vi "AlignProc.vi"(10 "BCGT":T1={"Brightness"=171.0, "Contrast"=89.0, "Gamma"=2.0, "Threshold_Low"=0.0, "Threshold_High"=144.0} {"Threshold_High" min=0.0 max=255.0 step=1.0 scale=0.0..255.0; "Threshold_Low" min=0 max=255 step=1 scale=0.0..255.0 scale format="%.2f"; "Gamma" min=0.1 max=10 step=0.01 scale=0.1..10.0 scale format="%.1f"; "Contrast" min=1 max=89 step=0.1 scale=0.0..89.0 scale format="%.2f"; "Brightness" min=0 max=255 step=1 scale=0.0..255.0 scale format="%.2f"}, 11 "Img_In":T2(plugin-control)) -> (0 "Distances":sgl[](array[numeric]) format="%.4f", 1 "Number of Particles":i32, 2 "Boolean":bool, 3 "Image Out":T2(plugin-control), 4 "Array":cluster{"Numeric":dbl, "Numeric":dbl}[](array[cluster]))   [LabVIEW 2013]
uses:
  <vilib>/Analysis/baseanly.llb/Mean (DBL).vi
  <vilib>/Analysis/NI_AALBase.lvlib
  <vilib>/vision/NI_Vision_Development_Module.lvlib
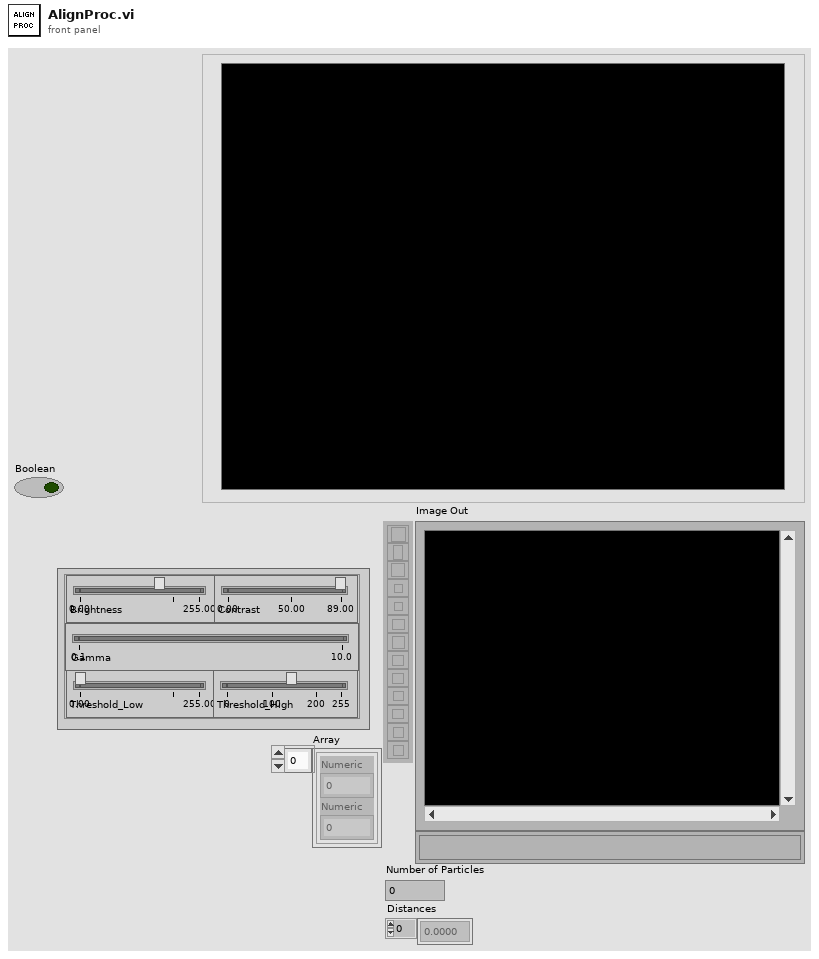
[diagram p1: front panel]
types:
  T1 = cluster{"Brightness":sgl, "Contrast":sgl, "Gamma":sgl, "Threshold_Low":sgl, "Threshold_High":dbl}
  T2 = typedef "IMAQ Image.ctl" = refnum<image>
  T3 = cluster{"Brightness":sgl, "Contrast":sgl, "Gamma":sgl}
  T4 = cluster{"Threshold_Low":sgl, "Threshold_High":dbl}
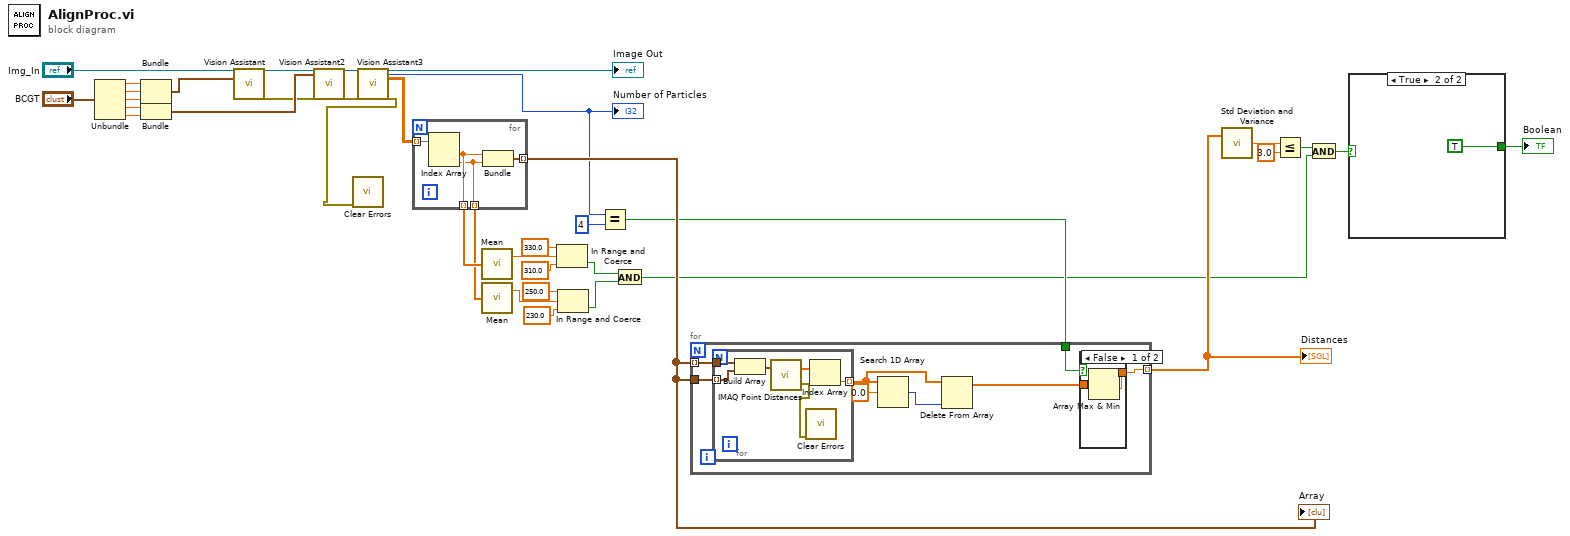
[diagram p0: block diagram]
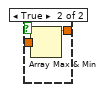
[diagram p2: hidden frame]
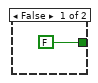
[diagram p3: hidden frame]
diagram:
  n1 = Unbundle("BCGT") -> ("Brightness"=w35:sgl, "Contrast"=w34:sgl, "Gamma"=w33:sgl, "Threshold_Low"=w31:sgl, "Threshold_High"=w30:dbl)
  n2 = Bundle("Brightness"=w35, "Contrast"=w34, "Gamma"=w33) -> (w32:T3)  [unwired: 1 in]
  n3 = Bundle("Threshold_Low"=w31, "Threshold_High"=w30) -> (w28:T4)  [unwired: 1 in]
  n4 = call "Vision Assistant"("Image In"="Img_In", "BCG Values (Brightness 1)"=w32) -> ("Image Out"=w29:T2, "error out"=w3:errorcluster)  [unwired: 24 in]
  n5 = call "Vision Assistant2"("Image In"=w29, "Range (Threshold 1)"=w28, "error in"=w3) -> ("Image Out"=w27:T2, "error out"=w2:errorcluster)  [unwired: 23 in]
  n6 = call "Vision Assistant3"("Image In"=w27, "error in"=w2) -> ("Image Out"=→"Image Out":T2, "Number of Particles (Particle Analysis 1)"=w19:i32, "Particle Measurements (Pixels) (Particle Analysis 1)"=w22:dbl[][], "error out"=w1:errorcluster)  [unwired: 22 in]
  "Number of Particles" <- w19
  n7 = call <vilib>:"Clear Errors.vi"("error in (no error)"=w1) -> ()  [unwired: 6 in, 1 out]
  n8 = for {
    tunnel: w22 -> [w41] mode=indexing
    tunnel: [w40] -> w20 mode=indexing
    tunnel: [w39] -> w14 mode=indexing
    tunnel: [w38] -> w13 mode=indexing
    n9 = Index Array(array=w41) -> (element #1=w39:dbl, element #2=w38:dbl)  [unwired: 2 in]
    n10 = Bundle("Numeric"=w39, "Numeric"=w38) -> (w40:cluster{"Numeric":dbl, "Numeric":dbl})  [unwired: 1 in]
  }
  "Array" <- w20
  n11 = call-poly <vilib>:"Mean.vi"("X"=w14) -> ("mean"=w12:dbl)  [unwired: 1 out]
  n12 = call-poly <vilib>:"Mean.vi"("X"=w13) -> ("mean"=w9:dbl)  [unwired: 1 out]
  n13 = In Range and Coerce(upper limit=330.0, x=w12, lower limit=310.0) -> (In Range?=w6:bool)  [unwired: 1 out]
  n14 = In Range and Coerce(upper limit=250.0, x=w9, lower limit=230.0 ("upper limit")) -> (In Range?=w5:bool)  [unwired: 1 out]
  n15 = Equal?(x=w19, y=4) -> (x = y?=w17:bool)
  n16 = And(x=w6, y=w5) -> (x .and. y?=w4:bool)
  n17 = for {
    tunnel: w20 -> [w49] mode=indexing
    tunnel: w20 -> [w48]
    tunnel: [w47] -> w21 mode=indexing
    tunnel: w17 -> [w46]
    n18 = for {
      tunnel: w49 -> [w59]
      tunnel: w48 -> [w58] mode=indexing
      tunnel: [w55] -> w44 mode=indexing
      n19 = Build Array(w59, w58) -> (w57:cluster{"Numeric":dbl, "Numeric":dbl}[])
      n20 = call "IMAQ Point Distances"("Points"=w57) -> ("Distances"=w56:sgl[], "error out"=w54:errorcluster)  [unwired: 4 in]
      n21 = call <vilib>:"Clear Errors.vi"("error in (no error)"=w54) -> ()  [unwired: 6 in, 1 out]
      n22 = Index Array(array=w56) -> (element=w55:sgl)  [unwired: 1 in]
    }
    n23 = Search 1D Array(1D array=w44, element=sgl 0.0) -> (index of element=w43:i32)  [unwired: 1 in]
    n24 = Delete From Array(array=w44, index=w43) -> (array with subset deleted=w42:sgl[])  [unwired: 1 in, 1 out]
    n25 = case shown="False" w46 {
      tunnel: w42 -> [w51 w53]
      tunnel: [w50 w52] -> w47
      frame False {
        n26 = Array Max & Min(array=w51) -> (min value=w50:sgl)  [unwired: 3 out]
      }
      frame True {
        n27 = Array Max & Min(array=w53) -> (max value=w52:sgl)  [unwired: 3 out]
      }
    }
  }
  "Distances" <- w21
  n28 = call <vilib>:"Std Deviation and Variance.vi"("X"=w21) -> ("standard deviation"=w25:dbl)  [unwired: 1 in, 2 out]
  n29 = Less Or Equal?(x=w25, y=3.0) -> (x <= y?=w16:bool)
  n30 = And(x=w16, y=w4) -> (x .and. y?=w15:bool)
  n31 = case shown="True" w15 {
    tunnel: [FALSE TRUE] -> w23
    frame False {
    }
    frame True {
    }
  }
  "Boolean" <- w23
